vi "DEMO.vi"() -> ()   [LabVIEW 2012, in "Array FIFO.lvlib"]
uses:
  Array FIFO.lvlib
panel:
  out "波形图":dbl[](graph)
  in  "停止":bool
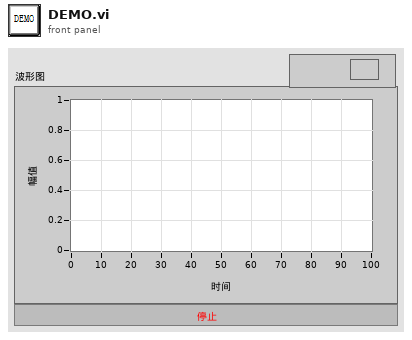
[diagram p1: front panel]
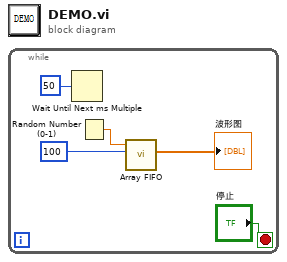
[diagram p0: block diagram]
diagram:
  n1 = while {
    stop <- "停止" stop-if-true
    n2 = Wait Until Next ms Multiple(millisecond multiple=u32 50 ("毫秒倍数")) -> ()  [unwired: 1 out]
    n3 = Random Number (0-1)() -> (number: 0 to 1=w2:dbl)
    n4 = call-poly "Array FIFO.vi"("length"=100, "input"=w2) -> ("Current Queue"=→"波形图":dbl[])  [unwired: 6 in, 3 out]
  }
